vi "Write.vi"(8 "error in (no error)":errorcluster, 10 "Data Class Array":refnum<class "Data Class.lvclass">[](array[class]), 11 "Data Class Array in":refnum<class "Data Class Array.lvclass">) -> (0 "error out":errorcluster, 1 "Success?":bool, 3 "Data Class Array out":refnum<class "Data Class Array.lvclass">)   [LabVIEW 2020, in "Data.lvlib" / "Data Class Array.lvclass"]
doc: "Write Data Class Array."
uses:
  Data Class Array.lvclass
  Data Class/Data Class.lvclass
  C:/Users/Henri/OneDrive/LabVIEW/Framework/Data/Data.lvclass
  Data Class Array.lvclass/Data Class Array.ctl
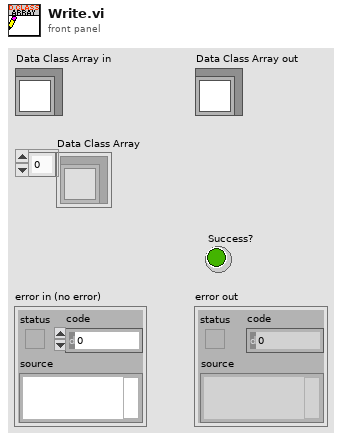
[diagram p1: front panel]
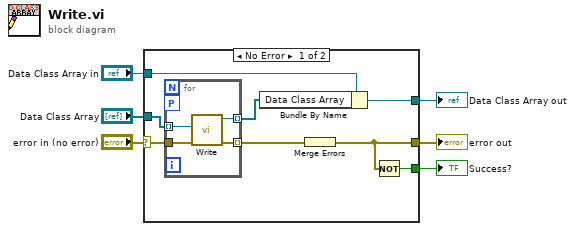
[diagram p0: block diagram]
diagram:
  n1 = case shown="No Error" "error in (no error)" {
    selector: "error in (no error)" -> [w10 w19]
    tunnel: [w7 w19] -> w6
    tunnel: [w13 w20] -> w4
    tunnel: "Data Class Array in" -> [w14 w20]
    tunnel: "Data Class Array" -> [w12 _]
    tunnel: [w8 _] -> w3
    frame No Error {
      n2 = for {
        tunnel: w12 -> [w17] mode=indexing
        tunnel: [w15] -> w11 mode=indexing
        tunnel: w10 -> [w16]
        tunnel: [w18] -> w9 mode=indexing
        workers-P: _ -> [_]
        n3 = call "Write.vi"("error in (no error)"=w16, "Data"=w17) -> ("error out"=w18:errorcluster, "Data Class out"=w15:refnum<class "Data Class.lvclass">)  [unwired: 8 in]
      }
      n4 = Bundle By Name(cluster=w14, "Data Class Array"=w11) -> (w13:refnum<class "Data Class Array.lvclass">)
      n5 = Merge Errors(w9) -> (w7:errorcluster)
      n6 = Not(x=w7) -> (.not. x?=w8:bool)
    }
    frame Error {
    }
  }
  "error out" <- w6
  "Data Class Array out" <- w4
  "Success?" <- w3
